vi "Write Data to Caller.vi"(8 "error in (no error)":errorcluster, 11 "Data":string) -> (0 "error out":errorcluster)   [LabVIEW 2020]
uses:
  vi.lib/LabVIEW Icon API/lv_icon/lv_icon.lvlib
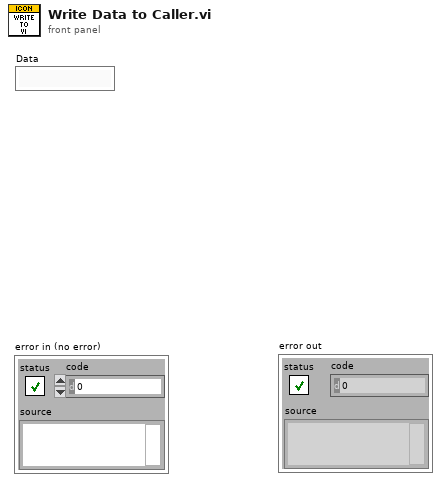
[diagram p1: front panel]
types:
  T1 = typedef "Who Invoked Icon Editor.ctl" = cluster{"Icon Editor Invoker Type":T2, "App Refnum of Invoker":refnum<vi>, "Qualified Name of Invoker":string, "Path to Invoker":path}
  T2 = typedef "Icon Editor Invoker Type.ctl" = enum32{"Unknown Icon Source", "VI Icon", "Library Icon (any library type)", "Palette icon", "Icon from App Method"}
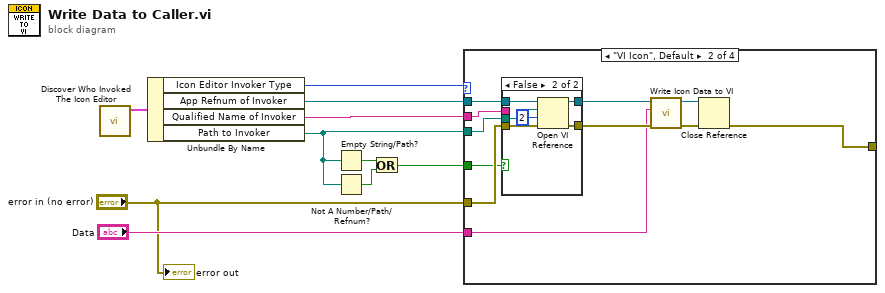
[diagram p0: block diagram]
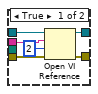
[diagram p3: hidden frame]
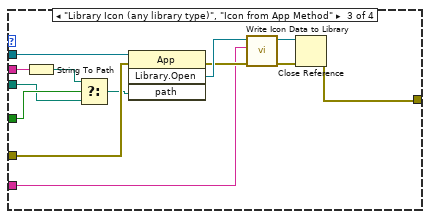
[diagram p4: hidden frame]
diagram:
  n1 = call <resource>:"Discover Who Invoked The Icon Editor.vi"() -> ("Who Invoked The Icon Editor?"=w10:T1)  [unwired: 11 out]
  n2 = Unbundle By Name(w10) -> ("Icon Editor Invoker Type"=w8:T2, "App Refnum of Invoker"=w9:refnum<vi>, "Qualified Name of Invoker"=w3:string, "Path to Invoker"=w2:path)
  n3 = Empty String/Path?(string/path=w2) -> (empty?=w5:bool)
  n4 = Not A Number/Path/Refnum?(number/path/refnum=w2) -> (NaN/Path/Refnum?=w4:bool)
  n5 = Or(x=w5, y=w4) -> (x .or. y?=w1:bool)
  n6 = case shown="\"VI Icon\", Default" w8 {
    tunnel: "error in (no error)" -> [w11 w22 w40 w48]
    tunnel: [w11 w17 w46 w48] -> _
    tunnel: w9 -> [_ w16 w47 _]
    tunnel: "Data" -> [_ w15 w41 _]
    tunnel: w3 -> [_ w13 w36 _]
    tunnel: w2 -> [_ w12 w38 _]
    tunnel: w1 -> [_ w14 w39 _]
    frame "Unknown Icon Source" {
    }
    frame "VI Icon", Default {
      n7 = case shown="False" w14 {
        tunnel: w22 -> [w28 w34]
        tunnel: [w27 w33] -> w21
        tunnel: [w26 w32] -> w20
        tunnel: w16 -> [w25 w31]
        tunnel: w13 -> [w24 _]
        tunnel: w12 -> [_ w30]
        frame True {
          n8 = Open VI Reference(application reference (local)=w25, vi path=w24, options=2, error in (no error)=w28) -> (vi reference=w27:refnum<vi>, error out=w26:errorcluster)  [unwired: 2 out]
        }
        frame False {
          n9 = Open VI Reference(application reference (local)=w31, vi path=w30, options=2, error in (no error)=w34) -> (vi reference=w33:refnum<vi>, error out=w32:errorcluster)  [unwired: 2 out]
        }
      }
      n10 = call "Write Icon Data to VI.vi"("error in (no error)"=w20, "Data"=w15, "VI Ref in"=w21) -> ("error out"=w18:errorcluster, "VI Ref out"=w19:refnum<vi>)  [unwired: 7 in]
      n11 = Close Reference(reference=w19, error in (no error)=w18) -> (error out=w17:errorcluster)
    }
    frame "Library Icon (any library type)", "Icon from App Method" {
      n12 = String To Path(string=w36) -> (path=w35:path)
      n13 = Select(t=w35, s=w39, f=w38) -> (s? t:f=w37:path)
      n14 = invoke class="App" method="Library.Open"(reference=w47, error in=w40, "path"=w37) -> (error out=w44:errorcluster, "Open Library"=w45:refnum<vi>)  [unwired: 1 in, 2 out]
      n15 = call "Write Icon Data to Library.vi"("error in (no error)"=w44, "Data"=w41, "Library Ref in"=w45) -> ("error out"=w43:errorcluster, "Library Ref out"=w42:refnum<vi>)  [unwired: 7 in]
      n16 = Close Reference(reference=w42, error in (no error)=w43) -> (error out=w46:errorcluster)
    }
    frame "Palette icon" {
    }
  }
  "error out" <- "error in (no error)"
